vi "Get_PackedLibrary_Data.vi"(8 "error in (no error)":errorcluster, 11 "Class in":refnum<class "AB_PackedLibrary.lvclass">) -> (0 "error out":errorcluster, 2 "data":T1, 3 "Class out":refnum<class "AB_PackedLibrary.lvclass">)   [LabVIEW 2020, in "AB_PackedLibrary.lvclass"]
uses:
  <vilib>/AppBuilder/AB_Classes/PackedLib/AB_PackedLibrary.lvclass
  <vilib>/AppBuilder/AB_Classes/PackedLib/AB_PackedLibrary.ctl
  <vilib>/AppBuilder/AB_Classes/PackedLib/AB_PackedLibrary.lvclass/AB_PackedLibrary.ctl
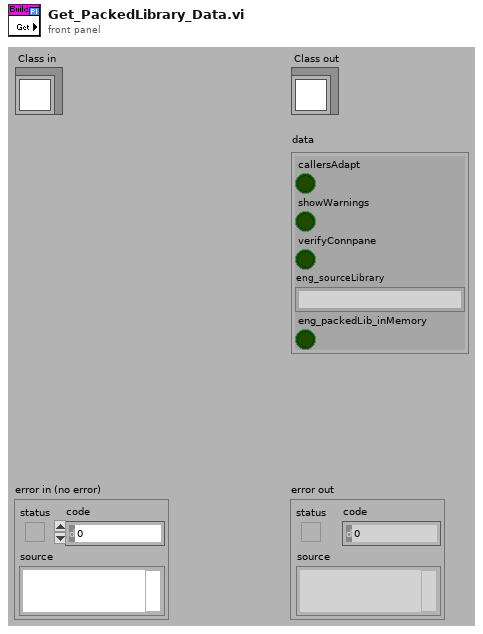
[diagram p1: front panel]
types:
  T1 = typedef "AB_PackedLibrary.ctl" = cluster{"callersAdapt":bool, "showWarnings":bool, "verifyConnpane":bool, "eng_sourceLibrary":string, "eng_packedLib_inMemory":bool}
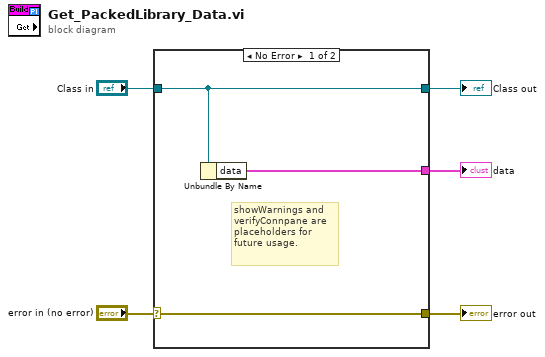
[diagram p0: block diagram]
diagram:
  n1 = case shown="No Error" "error in (no error)" {
    selector: "error in (no error)" -> [w8 w10]
    tunnel: [w8 w10] -> w4
    tunnel: [w7 w9] -> w2
    tunnel: "Class in" -> [w7 w9]
    tunnel: [w6 _] -> w1
    frame No Error {
      # "showWarnings and verifyConnpane are placeholders for future usage."
      n2 = Unbundle By Name(w7) -> ("data"=w6:T1)
    }
    frame Error {
    }
  }
  "Class out" <- w2
  "error out" <- w4
  "data" <- w1
